vi "dummy.vi"(8 "error in (no error)":errorcluster, 11 "ICSettingsViewer in":refnum<class "ICSettingsViewer.lvclass">) -> (0 "error out":errorcluster, 3 "ICSettingsViewer out":refnum<class "ICSettingsViewer.lvclass">)   [LabVIEW 2009, in "Views.lvlib" / "Camera.lvlib" / "ICSettingsViewer.lvclass"]
uses:
  ICSettingsViewer.lvclass
  Tools/SettingsEventManager/SettingsEventsManager.lvclass
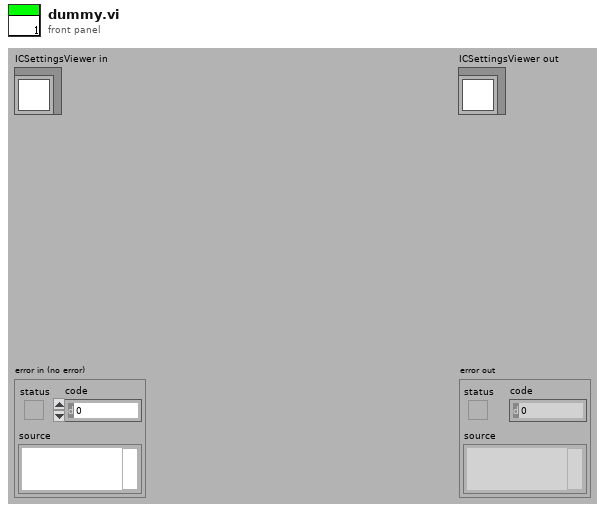
[diagram p1: front panel]
types:
  T1 = cluster{"settingsFrontEndEvents":cluster{"loadSettingsFromPath":refnum<user-event>, "lookUpElementEvent":refnum<user-event>, "saveSettings":refnum<user-event>, "loadSettings":refnum<user-event>, "close":refnum<user-event>, "replaceElement":refnum<user-event>, "findParentNodes":refnum<user-event>, "createNode":refnum<user-event>}, "settingBackEndEvents":cluster{"defaultSettingsPathRequest":refnum<user-event>, "searchResultEvent":refnum<user-event>, "settingsSaved":refnum<user-event>, "settingsLoaded":refnum<user-event>, "foundParentNode":refnum<user-event>}}
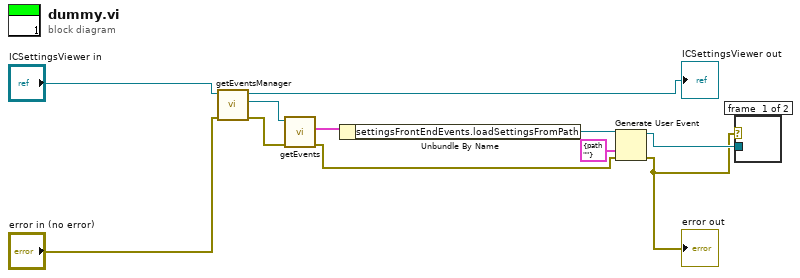
[diagram p0: block diagram]
diagram:
  n1 = call-dynamic "getEventsManager.vi"("error in (no error)"="error in (no error)", "SettingsViewer.lvclass in"="ICSettingsViewer in") -> ("error out"=w3:errorcluster, "Tools.lvlib:Settings.lvlib:SettingsEventsManager.lvclass"=w9:refnum<class "SettingsEventsManager.lvclass">, "SettingsViewer.lvclass out"=→"ICSettingsViewer out":refnum<class "ICSettingsViewer.lvclass">)  [unwired: 7 in]
  n2 = call-dynamic "getEvents.vi"("error in (no error)"=w3, "SettingsEventsManager in"=w9) -> ("error out"=w4:errorcluster, "settingsEvents"=w8:T1)  [unwired: 7 in, 1 out]
  n3 = Unbundle By Name(w8) -> ("settingsFrontEndEvents.loadSettingsFromPath"=w7:refnum<user-event>)
  n4 = Generate User Event(user event=w7, event data cluster=cluster{"Path":path} {"Path"=path ""} ("event data"), error in=w4) -> (user event out=w2:refnum<user-event>, error out=w1:errorcluster)
  "error out" <- w1
  n5 = case shown="No Error" w1 {
    tunnel: w2 -> [_ _]
    frame #0 {
    }
    frame #1 {
    }
  }
